vi "Receive ILC Inputs.vi"(8 "error in (no error)":errorcluster, 11 "Model in":refnum<class "Model.lvclass">) -> (0 "error out":errorcluster, 3 "Model out":refnum<class "Model.lvclass">)   [LabVIEW 2015, in "Model.lvclass"]
uses:
  Model.lvclass
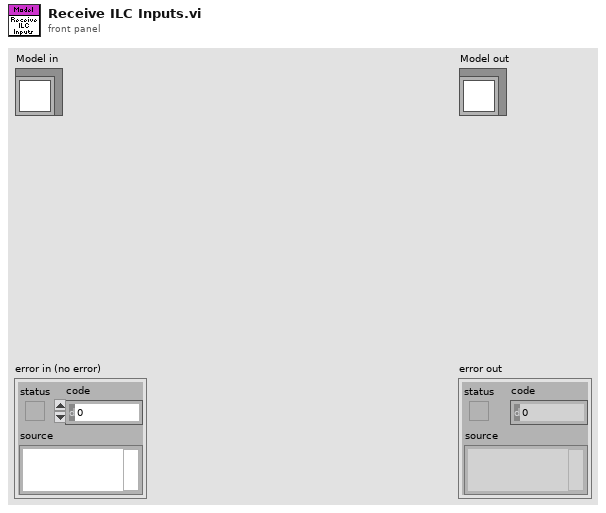
[diagram p1: front panel]
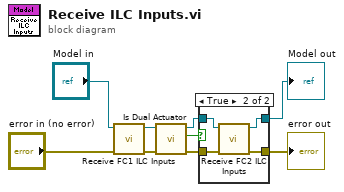
[diagram p0: block diagram]
diagram:
  n1 = call "Receive FC1 ILC Inputs.vi"("error in (no error)"="error in (no error)", "Model in"="Model in") -> ("error out"=w4:errorcluster, "Model out"=w5:refnum<class "Model.lvclass">)  [unwired: 8 in]
  n2 = call "Is Dual Actuator.vi"("error in (no error)"=w4, "Model in"=w5) -> ("error out"=w3:errorcluster, "Is Dual Actuator"=w2:bool, "Model out"=w1:refnum<class "Model.lvclass">)  [unwired: 7 in]
  n3 = case shown="True" w2 {
    tunnel: w1 -> [w11 w15]
    tunnel: [w11 w14] -> w8
    tunnel: [w10 w13] -> w7
    tunnel: w3 -> [w10 w12]
    frame False {
    }
    frame True {
      n4 = call "Receive FC2 ILC Inputs.vi"("error in (no error)"=w12, "Model in"=w15) -> ("error out"=w13:errorcluster, "Model out"=w14:refnum<class "Model.lvclass">)  [unwired: 8 in]
    }
  }
  "error out" <- w7
  "Model out" <- w8
